vi "getCategoryAmount.vi"(8 "error in (no error)":errorcluster, 10 "Category.lvclass":refnum<class "Category.lvclass">, 11 "Account History in":refnum<class "Account History.lvclass">) -> (0 "error out":errorcluster, 2 "Default Amount":dbl, 3 "Account History out":refnum<class "Account History.lvclass">)   [LabVIEW 2018, in "Account History.lvclass"]
uses:
  Account History.lvclass
  Category/Category.lvclass
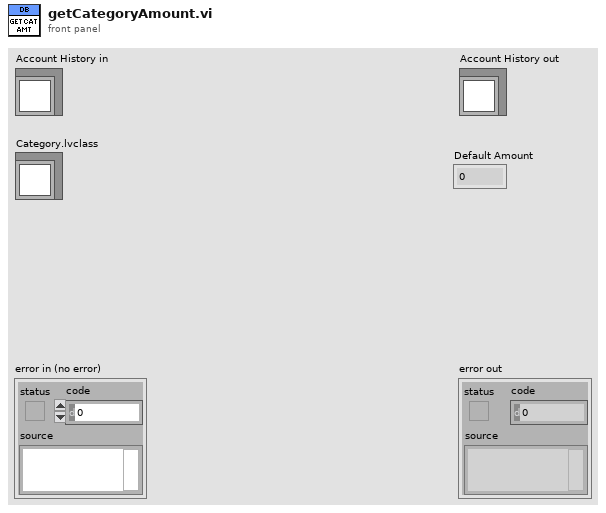
[diagram p1: front panel]
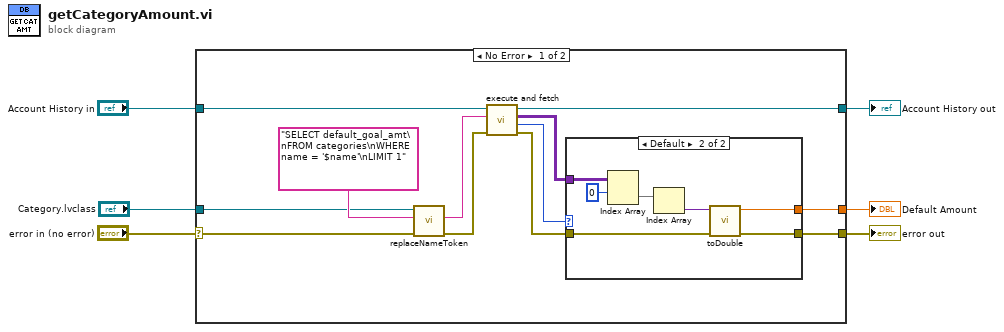
[diagram p0: block diagram]
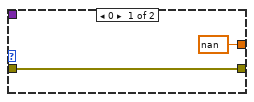
[diagram p2: hidden frame]
diagram:
  n1 = case shown="No Error" "error in (no error)" {
    selector: "error in (no error)" -> [w8 w29]
    tunnel: [w12 w29] -> w5
    tunnel: [w14 w28] -> w3
    tunnel: "Account History in" -> [w15 w28]
    tunnel: [w13 _] -> w2
    tunnel: "Category.lvclass" -> [w7 _]
    frame No Error {
      n2 = call "replaceNameToken.vi"("error in (no error)"=w8, "Query In"="SELECT default_goal_amt\nFROM categories\nWHERE name = '$name'\nLIMIT 1", "Category in"=w7) -> ("error out"=w11:errorcluster, "Query Out"=w10:string)  [unwired: 6 in, 1 out]
      n3 = call "execute and fetch.vi"("error in (no error)"=w11, "SQL query"=w10, "Database in"=w15) -> ("error out"=w17:errorcluster, "Num records"=w16:i32, "recordset data"=w18:variant[][], "Database out"=w14:refnum<class "Account History.lvclass">)  [unwired: 5 in]
      n4 = case shown="Default" w16 {
        tunnel: w18 -> [_ w27]
        tunnel: w17 -> [w20 w23]
        tunnel: [nan ("type") w22] -> w13
        tunnel: [w20 w21] -> w12
        frame 0 {
        }
        frame Default {
          n5 = Index Array(array=w27, index (row)=0) -> (element=w25:variant[])  [unwired: 1 in]
          n6 = Index Array(array=w25) -> (element=w24:variant)  [unwired: 1 in]
          n7 = call "toDouble.vi"("error in (no error)"=w23, "Value"=w24) -> ("error out"=w21:errorcluster, "type"=w22:dbl)  [unwired: 8 in]
        }
      }
    }
    frame Error {
    }
  }
  "error out" <- w5
  "Account History out" <- w3
  "Default Amount" <- w2
